vi "Tree Columns.vi"() -> (1 "Column Widths":i32[](array[numeric])=[300, 180, 60, 60, 60, 70, 110, 70, 70, 70, 450], 2 "Column Data Type":enum16{"String", "Numeric"}[](array[ring]), 3 "Column Labels":string[](array[string])=["VI Name", "State", "Reentrant", "Reentrancy Type", "FP Behavior", "Code Size", "Data Size", "VI Path"], 4 "Columns Updated Dynamically":i32[](array[numeric])=[2, 3, 4, 5, 8])   [LabVIEW 2013, in "LVTM.lvlib"]
uses:
  LVTM.lvlib
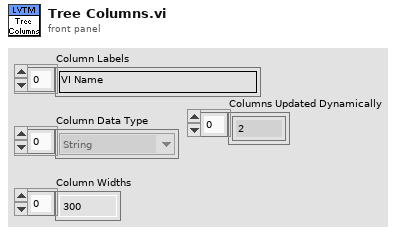
[diagram p1: front panel]
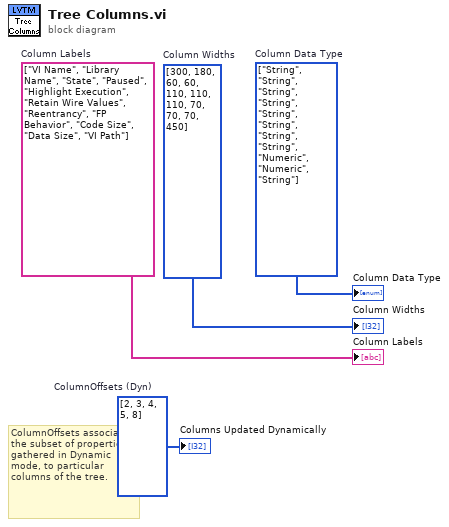
[diagram p0: block diagram]
diagram:
  w1 = i32[] [2, 3, 4, 5, 8]  # ColumnOffsets (Dyn)
  w4 = i32[] [300, 180, 60, 60, 110, 110, 110, 70, 70, 70, 450]  # Column Widths
  w3 = enum16{"String", "Numeric"}[] [enum."String", enum."String", enum."String", enum."String", enum."String", enum."String", enum."String", enum."String", enum."Numeric", enum."Numeric", enum."String"] items=["String", "Numeric"]  # Column Data Type
  w2 = string[] ["VI Name", "Library Name", "State", "Paused", "Highlight Execution", "Retain Wire Values", "Reentrancy", "FP Behavior", "Code Size", "Data Size", "VI Path"]  # Column Labels
  # "ColumnOffsets associates the subset of properties, gathered in Dynamic mode, to particular columns of the tree."
  "Column Labels" <- w2
  "Column Data Type" <- w3
  "Column Widths" <- w4
  "Columns Updated Dynamically" <- w1
